vi "API_GlobalMemoryStatus.vi"(8 "错误输入（无错误）":errorcluster) -> (0 "错误输出":errorcluster, 3 "memorystatus":T1)   [LabVIEW 2012, in "API.lvlib"]
uses:
  API.lvlib
  kernel32.dll
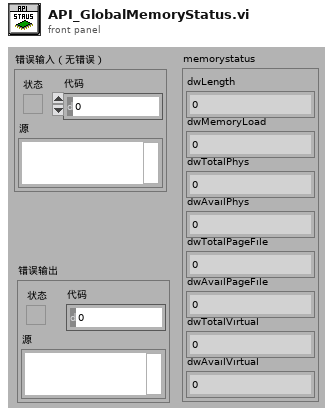
[diagram p1: front panel]
types:
  T1 = cluster{"dwLength":u32, "dwMemoryLoad":u32, "dwTotalPhys":u32, "dwAvailPhys":u32, "dwTotalPageFile":u32, "dwAvailPageFile":u32, "dwTotalVirtual":u32, "dwAvailVirtual":u32}
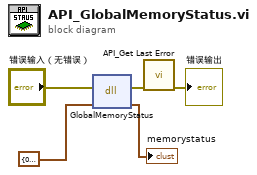
[diagram p0: block diagram]
diagram:
  n1 = dll-call lib="kernel32.dll" fn="GlobalMemoryStatus"(error in="错误输入（无错误）", "memorystatus"=T1 {"dwLength"=0, "dwMemoryLoad"=0, "dwTotalPhys"=0, "dwAvailPhys"=0, "dwTotalPageFile"=0, "dwAvailPageFile"=0, "dwTotalVirtual"=0, "dwAvailVirtual"=0}) -> (error out=w2:errorcluster, "memorystatus"=→"memorystatus":T1)  [unwired: 2 in, 2 out]
  n2 = call "API_Get Last Error.vi"("错误输入（无错误）"=w2) -> ("错误输出"=→"错误输出":errorcluster)  [unwired: 10 in]
